vi "CG test stand DAQ main V3 LJ.vi"() -> ()   [LabVIEW 2023]
doc: "This example demonstrates how to read N channels of analog input from a LINX device."
uses:
  <vilib>/MakerHub/LINX/Public/Peripherals/Digital/Digital Write N Chans.vi
  <vilib>/MakerHub/LINX/Public/Peripherals/Analog/Analog Read N Chans.vi
  <vilib>/MakerHub/LINX/Private/Local IO/LinxDigitalWrite.vi
  <vilib>/MakerHub/LINX/Public/Utilities/Check Channel.vi
  <vilib>/MakerHub/LINX/Private/Local IO/LinxAnalogRead.vi
  <vilib>/MakerHub/LINX/Public/Utilities/Open Serial.vi
  <vilib>/MakerHub/LINX/Private/Utilties/Generate Error.vi
  <vilib>/Analysis/Matrix/Numeric/Conversions/Array To Matrix - RA.vi
  <vilib>/Utility/file.llb/Write Delimited Spreadsheet (DBL).vi
  <vilib>/MakerHub/LINX/LMH-LINX.lvlib
  <vilib>/Analysis/Matrix/NI_Matrix.lvlib
panel:
  in  "EIO Analog Enable":bool[](array[boolean])=[FALSE, FALSE, FALSE, FALSE, FALSE, FALSE, FALSE, FALSE]
  in  "FIO Analog Enable":bool[](array[boolean])=[FALSE, FALSE, FALSE, FALSE, FALSE, FALSE, FALSE, FALSE]
  in  "?":bool
  in  "Path":path
  out "Full filepath":string
  in  "File extension":string
  in  "Filename":string
  in  "Cal Value":dbl
  out "Time":timestamp
  out "Filewriting Error":errorcluster
  in  "FIO6":bool
  in  "FIO7":bool
  in  "DAC0":dbl format="%.4f"
  in  "Serial Port":refnum<visa-resource-name>
  out "LabJack Error":string
  in  "Device Selector":bool
  out "LABJACK U3 Error":errorcluster
  in  "Stop Button":bool
  in  "?":T1(tab)
  out "A0 B":dbl
  out "A0 X1":dbl
  out "A0 X2":dbl
  out "A0 X3":dbl
  out "A0 scaled":dbl
  out "A0_Instrumentlabel":dbl
  out "A0_Voltage":dbl
  out "A1":dbl
  out "A1_Voltage":dbl
  out "A2":dbl
  out "A2_Voltage":dbl
  out "A3":dbl
  out "A3_Voltage":dbl
  out "A1_Instrumentlabel":string
  out "A2_Instrumentlabel":string
  out "A3_Instrumentlabel":string
  out "A0_Instrumentlabel 2":string
  out "A2 B":dbl caption="A0 B"
  out "A2 X3":dbl caption="A0 X3"
  out "A2 X2":dbl caption="A0 X2"
  out "A2 X1":dbl caption="A0 X1"
  out "A2 scaled":dbl caption="A0 scaled"
  out "A3 B":dbl caption="A0 B"
  out "A3 X3":dbl caption="A0 X3"
  out "A3 X2":dbl caption="A0 X2"
  out "A3 X1":dbl caption="A0 X1"
  out "A3 scaled":dbl caption="A0 scaled"
  out "A4":dbl
  out "A4_Voltage":dbl
  out "A4_Instrumentlabel":string
  out "A4 X3":dbl caption="A0 X3"
  out "A4 X2":dbl caption="A0 X2"
  out "A4 X1":dbl caption="A0 X1"
  out "A4 B":dbl caption="A0 B"
  out "A4 scaled":dbl caption="A0 scaled"
  out "A4 2":dbl
  out "A5_Voltage":dbl
  out "A4_Instrumentlabel 2":string
  out "A5 B":dbl caption="A0 B"
  out "A5 X3":dbl caption="A0 X3"
  out "A5 X2":dbl caption="A0 X2"
  out "A5 X1":dbl caption="A0 X1"
  out "A5 scaled":dbl caption="A0 scaled"
  out "A2 scaled 2":dbl caption="A0 scaled"
  out "A2 X1 2":dbl caption="A0 X1"
  out "A2 X2 2":dbl caption="A0 X2"
  out "A2 X3 2":dbl caption="A0 X3"
  out "A2 B 2":dbl caption="A0 B"
  in  "?":string
  in  "Analog Port":dbl
  out "PLOT 2":dbl(graph)
  in  "?":string
  in  "Analog Port":dbl
  out "PLOT 1":dbl(graph)
  in  "Analog Port":dbl
  in  "?":string
  out "PLOT 3":dbl(graph)
  in  "Analog Port":dbl
  in  "?":string
  out "PLOT 4":dbl(graph)
  out "PT3":dbl
  out "TM-DEV-RES":dbl
  out "TM3":dbl
  out "TM2":dbl
  out "TM1":dbl
  out "PT1":dbl
  in  "Tare":dbl
  in  "Port":dbl
  out "Measured Load":dbl
  out "Loadcell Voltage":dbl
  in  "?":bool
  # "."
  # "HOW TO USE THIS SOFTWARE"
  # "1. Select the DAQ device you are using\n2. If you are using Arduino, select the COM port you are using\n3. Start the software by pressing CTRL+R"
  # "Analog Inputs"
  # "X1*V^1+X2*V^2+X3*V^3+B"
  # "Analog Port"
  # "Voltage In"
  # "X3"
  # "X2"
  # "X1"
  # "B"
  # "Instrument name"
  # "Scaled Value"
  # "F"
  # "psi"
  # "F"
  # "psi"
  # "F"
  # "psi"
  # "V"
  # "g"
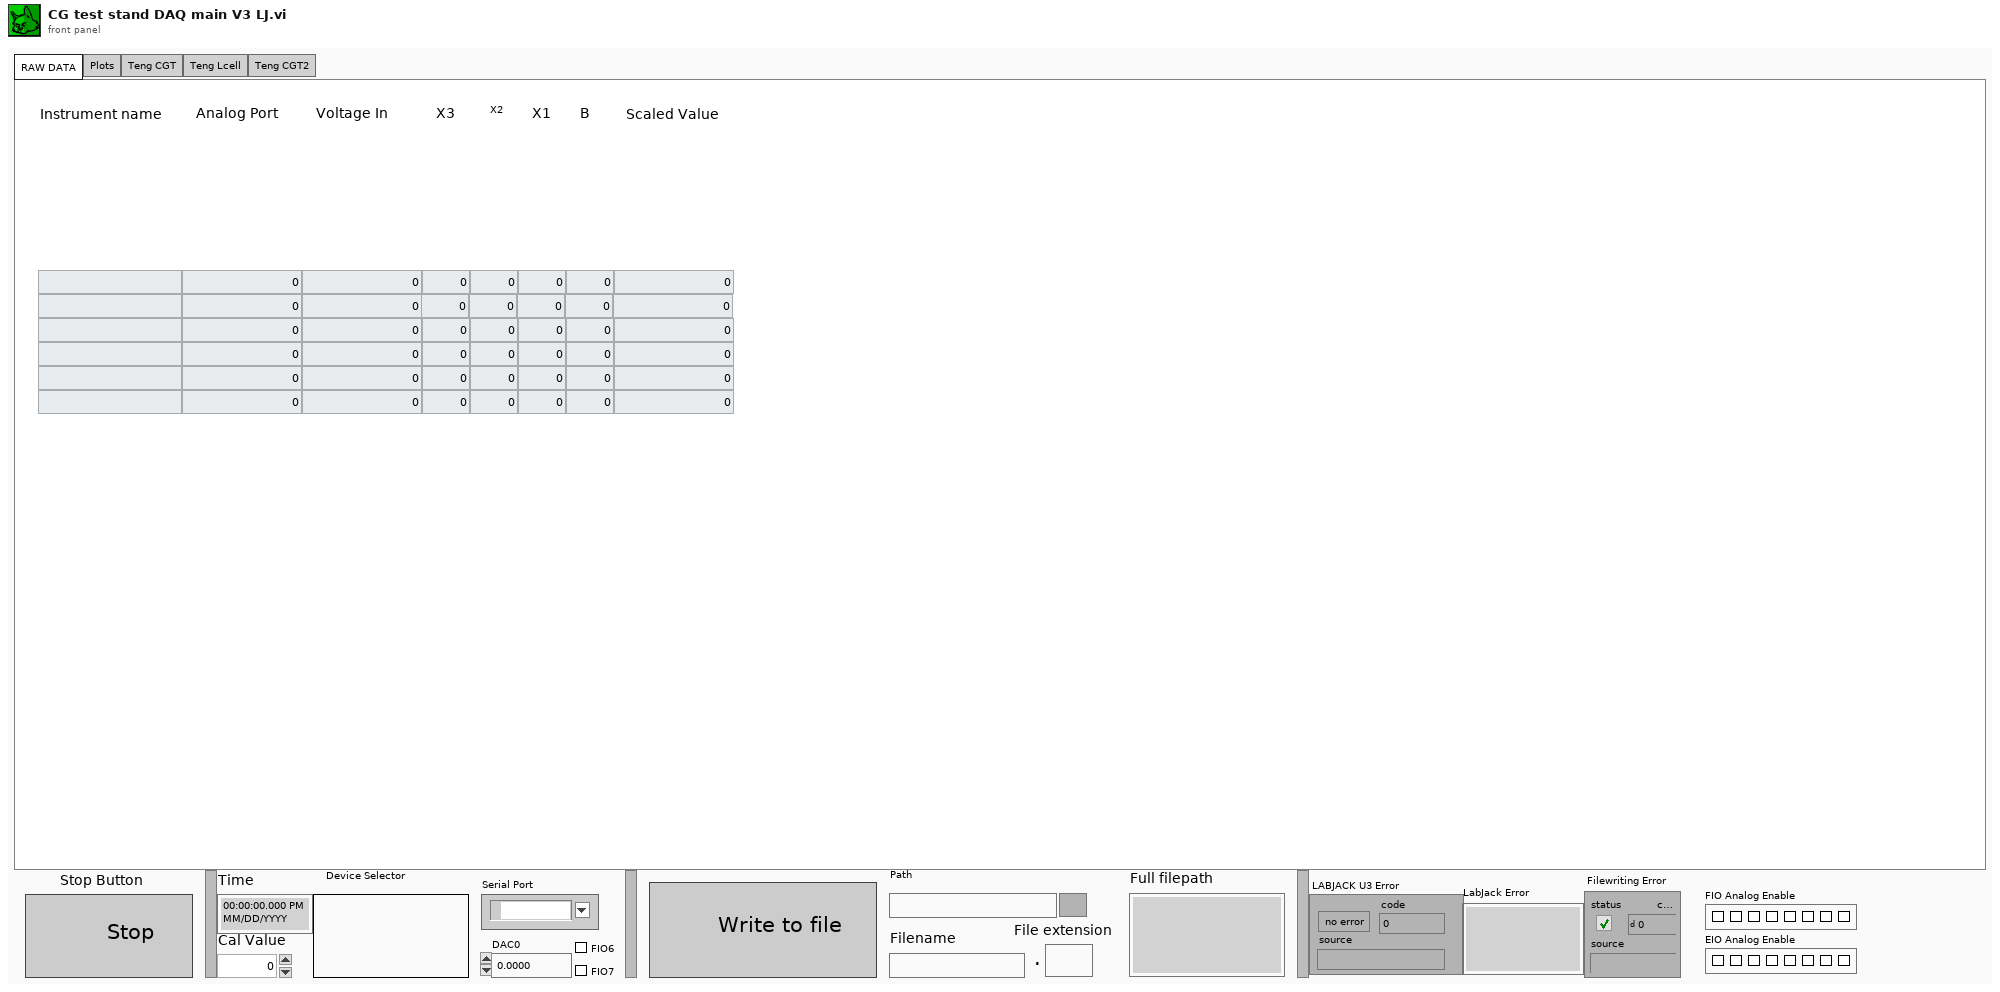
[diagram p1: front panel]
types:
  T1 = enum32{"RAW DATA", "Plots", "Teng CGT", "Teng Lcell", "Teng CGT2"}
  T2 = typedef "LMH-LINX.lvlib/LINX Ref.ctl" = cluster{"IO":T3, "Interface":T4, "LINX Device Config":T5}
  T3 = typedef "LMH-LINX.lvlib/Platform.ctl" = enum16{"Remote", "Local"}
  T4 = typedef "LMH-LINX.lvlib/Interface.ctl" = enum16{"Serial", "TCP"}
  T5 = typedef "LMH-LINX.lvlib/Device.lvlib/LINX Device Config.ctl" = cluster{"Interface":T4, "COM Port":refnum<visa-resource-name>, "TCP Configuration":T6, "Device Family":u8, "Device ID":u8, "Device Name":string, "TCP Ref":refnum<k5>, "Channels":T7}
  T6 = typedef "LMH-LINX.lvlib/Device.lvlib/TCP Config.ctl" = cluster{"IP Address":string, "Port":u16}
  T7 = typedef "LMH-LINX.lvlib/Channels.ctl" = cluster{"DI":u8[], "DO":u8[], "AI":u8[], "AO":u8[], "PWM":u8[], "QE":u8[], "UART":u8[], "I2C 2":u8[], "SPI":u8[], "CAN":u8[], "Servo":u8[], "AI Ref (V)":dbl, "AI Resolution (Bits)":u8, "AO Ref (V)":dbl, "AO Resolution (Bits)":u8}
  T8 = typedef "NI_Matrix.lvlib/RealMatrix.ctl" = dbl[][]
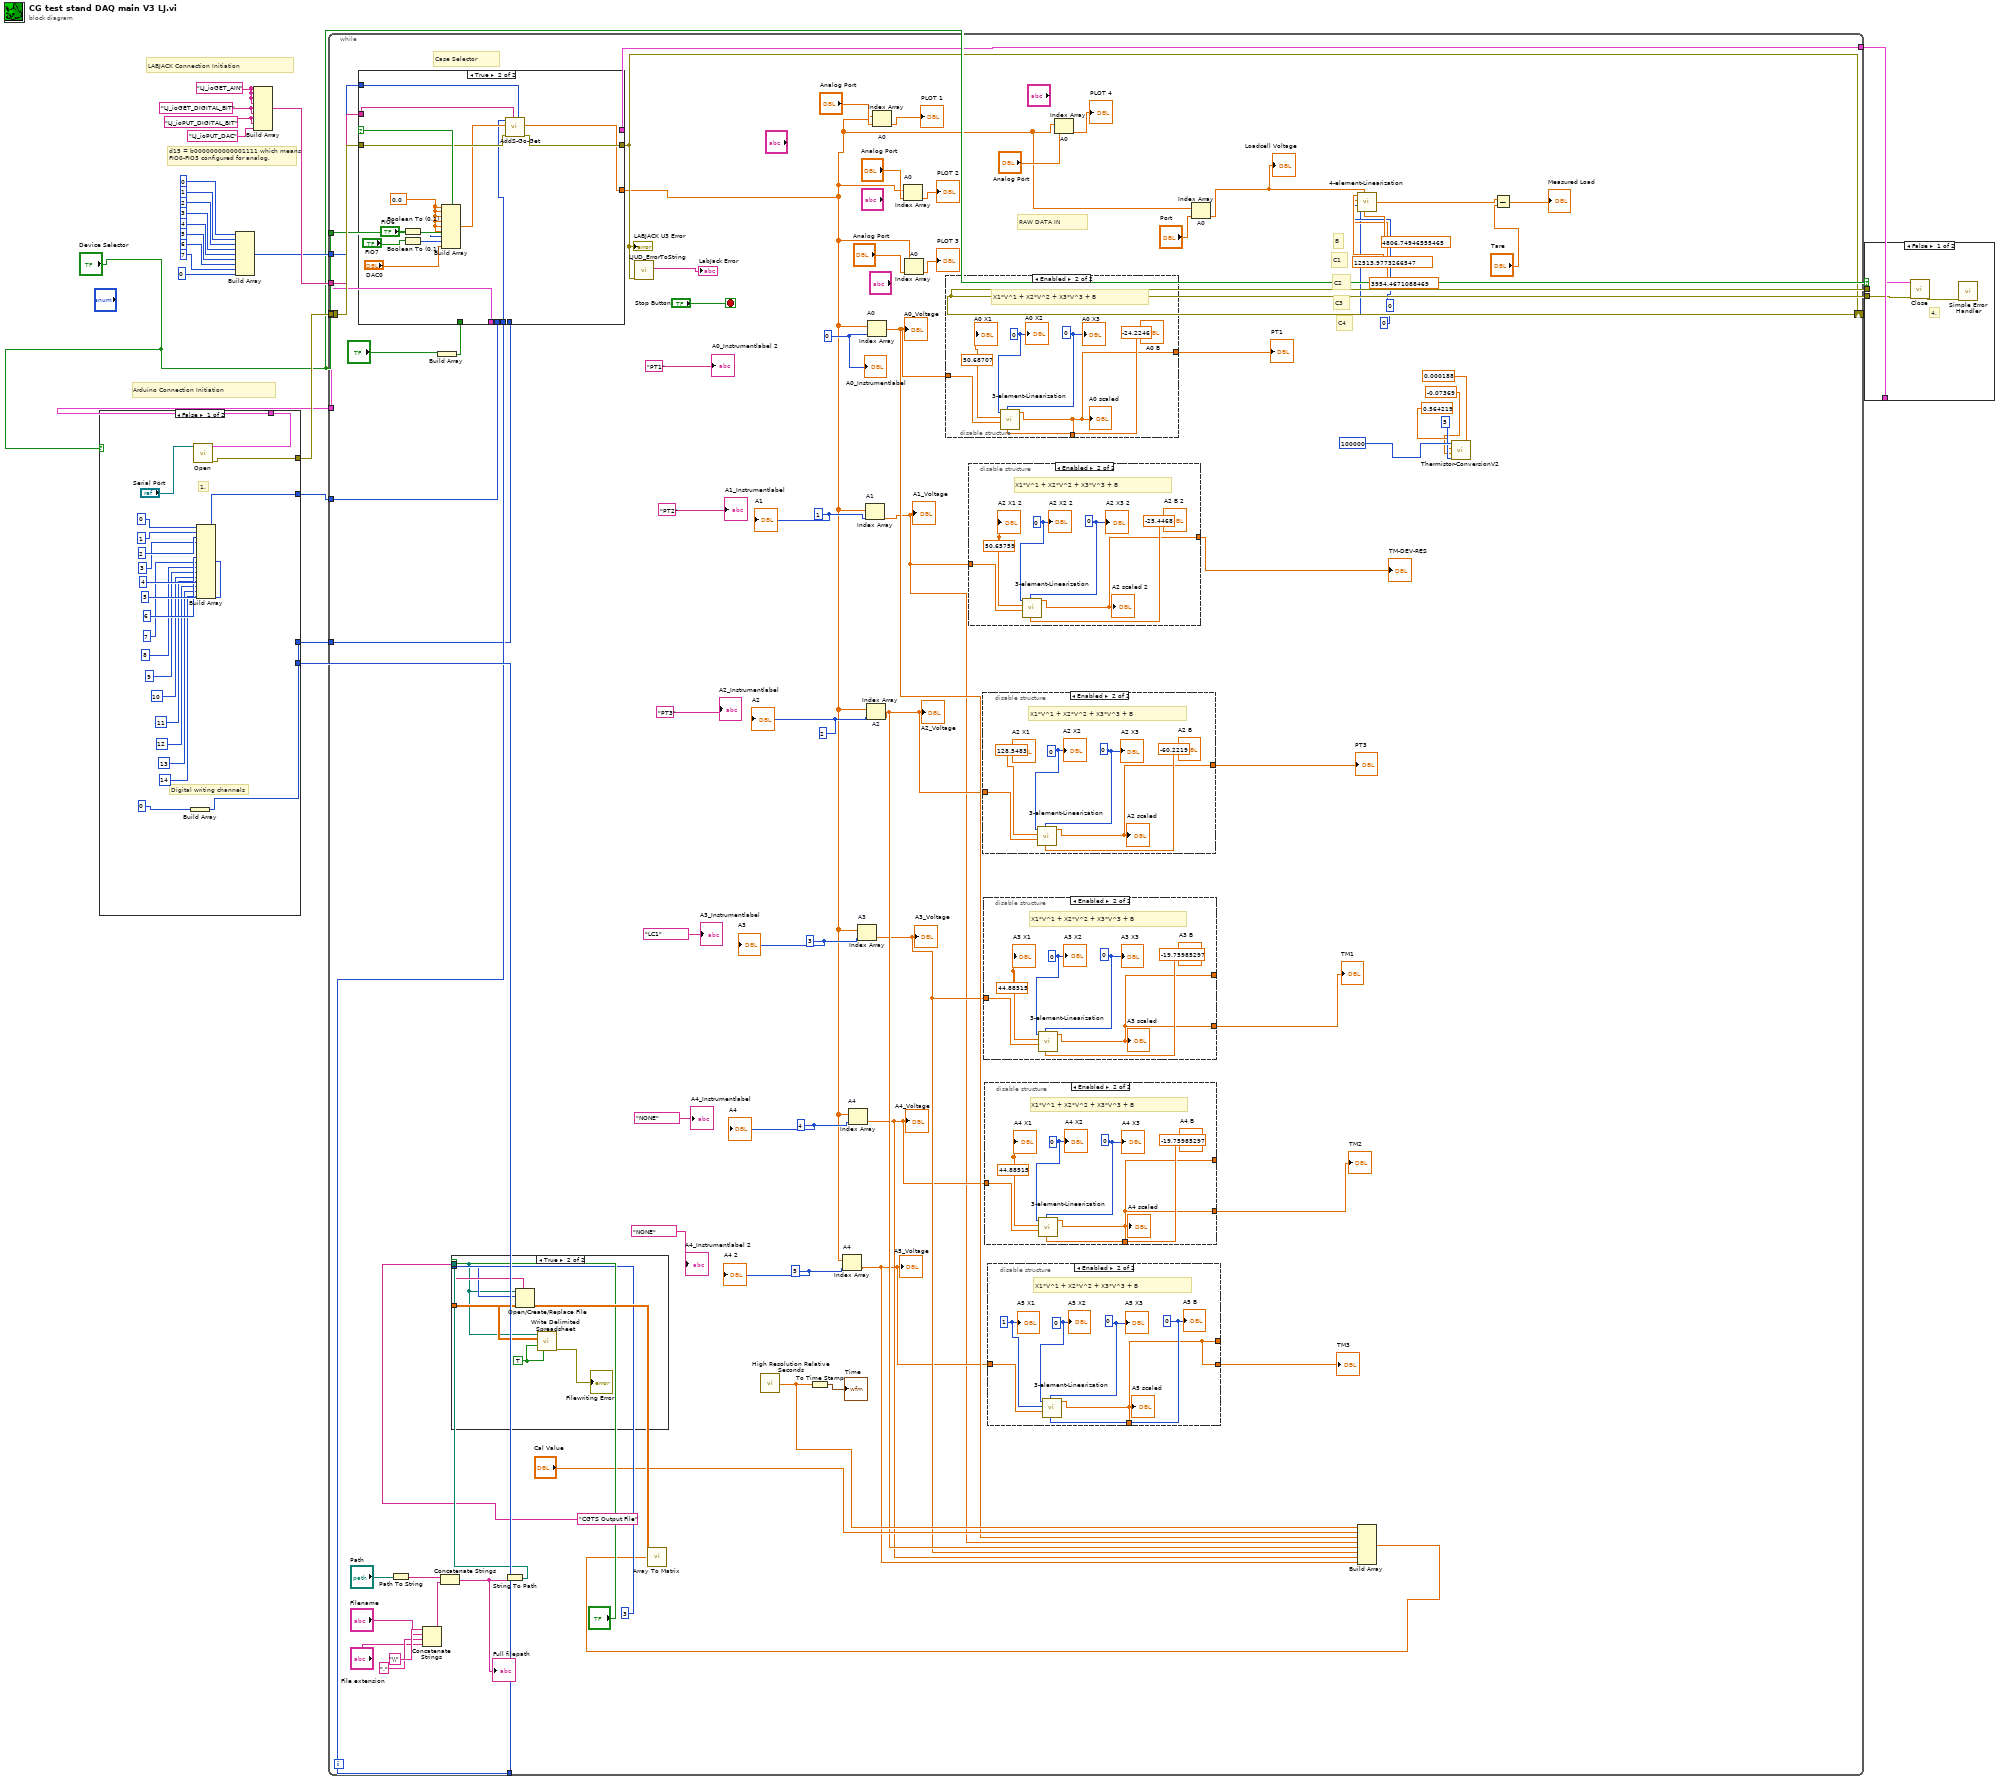
[diagram p0: block diagram]
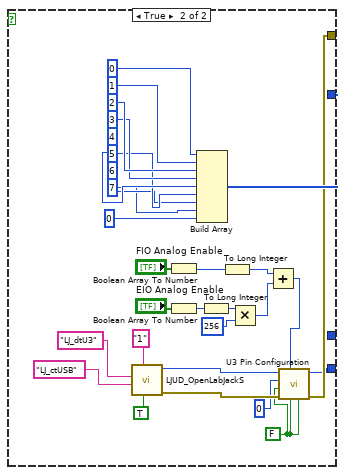
[diagram p3: hidden frame]
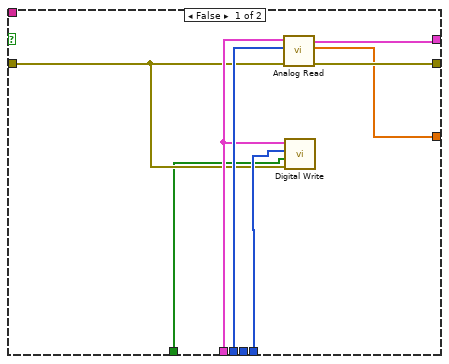
[diagram p11: hidden frame]
diagram:
  w21 = "LJ_ioPUT_DIGITAL_BIT" ("IOType")
  w23 = "LJ_ioGET_AIN" ("IOType")
  w22 = "LJ_ioGET_DIGITAL_BIT" ("IOType")
  # "Arduino Connection Initiation"
  # "LABJACK Connection Initiation"
  # "d15 = b0000000000001111 which means\nFIO0-FIO3 configured for analog."
  n1 = case shown="False" "Device Selector" {
    tunnel: [w38 w55] -> w19
    tunnel: [w37 _] -> w18
    tunnel: [w36 w64] -> w17
    tunnel: [_ w54] -> w3
    tunnel: [w33 _] -> w1
    frame False {
      # "Digital writing channels"
      # "1."
      n2 = Build Array(0) -> (w33:i32[])
      n3 = call-poly <vilib>:"Open.vi"("Serial Port"="Serial Port") -> ("Error Out"=w38:errorcluster, "LINX Resource"=w37:T2)  [unwired: 8 in, 1 out]
      n4 = Build Array(0, 1, 2, 3, 4, 5, 6, 7, 8, 9, 10, 11, 12, 13, 14) -> (w36:i32[])
    }
    frame True {
      w56 = FALSE ("Enable DAC1")
      n5 = call <vilib>:"LJUD_OpenLabJackS.vi"("FirstFound"=TRUE, "Address"="1", "ConnectionType"="LJ_ctUSB", "DeviceType"="LJ_dtU3") -> ("error out"=w59:errorcluster, "Handle"=w58:i32)  [unwired: 5 in, 1 out]
      n6 = Boolean Array To Number(Boolean array="FIO Analog Enable") -> (number=w49:u32)
      n7 = Boolean Array To Number(Boolean array="EIO Analog Enable") -> (number=w48:u32)
      n8 = Build Array(0, 1, 2, 3, 4, 5, 6, 7, 0) -> (w64:i32[])
      n9 = To Long Integer(number=w48) -> (32bit integer=w50:i32)
      n10 = To Long Integer(number=w49) -> (32bit integer=w47:i32)
      n11 = Multiply(x=w50, y=256) -> (x*y=w46:i32)
      n12 = Add(x=w47, y=w46) -> (x+y=w45:i32)
      n13 = call <vilib>:"U3 Pin Configuration.vi"("Enable Counter1"=w56, "Enable Counter0"=w56, "FIO/EIO Analog Enable"=w45, "error in"=w59, "Enable DAC1"=w56, "Number of Timers Enabled"=u8 0, "Handle In"=w58) -> ("error out"=w55:errorcluster, "Handle Out"=w54:i32)  [unwired: 3 in]
    }
  }
  n14 = Build Array(0, 1, 2, 3, 4, 5, 6, 7, 0) -> (w6:i32[])
  n15 = Build Array(w23, w23, w23, w23, w22, w22, w21, w21, "LJ_ioPUT_DAC" ("IOType")) -> (w16:string[])
  n16 = while {
    tunnel: w19 -> [w152]
    tunnel: w18 -> [w151]
    tunnel: [w150] -> w4
    shift-right: [w142] -> w5
    shift-left: _ -> [_]
    tunnel: w17 -> [w149]
    tunnel: "Device Selector" -> [w148]
    tunnel: w16 -> [w147]
    tunnel: w6 -> [w146]
    tunnel: w3 -> [w144]
    tunnel: w1 -> [w76]
    stop <- "Stop Button" stop-if-true
    w117 = 5
    w119 = 4
    w139 = 3
    w138 = 2
    w140 = 1
    w141 = 0
    # "B"
    # "C4"
    # "C3"
    # "C2"
    # "C1"
    # "RAW DATA IN"
    # "Case Selector"
    n17 = Path To String(path="Path") -> (string=w126:string)
    n18 = Concatenate Strings("\\", "Filename", ".", "File extension") -> (w125:string)
    n19 = Build Array("?") -> (w74:bool[])
    n20 = case shown="True" w148 {
      tunnel: [w202 w214] -> w142
      tunnel: w152 -> [w196 w215]
      tunnel: w151 -> [w198 _]
      tunnel: [w201 _] -> w150
      tunnel: w149 -> [w200 _]
      tunnel: w147 -> [_ w208]
      tunnel: w146 -> [_ w207]
      tunnel: [w199 w204] -> w102
      tunnel: w144 -> [_ w203]
      tunnel: w76 -> [w197 _]
      tunnel: w74 -> [w195 _]
      frame False {
        n21 = call-poly <vilib>:"Analog Read.vi"("Error In"=w196, "AI Channel(s)"=w200, "LINX Resource"=w198) -> ("Error Out"=w202:errorcluster, "Voltages"=w199:dbl[], "LINX Resource"=w201:T2)  [unwired: 5 in, 1 out]
        n22 = call-poly <vilib>:"Digital Write.vi"("Error In"=w196, "Values"=w195, "DO Channels"=w197, "LINX Resource"=w198) -> ()  [unwired: 6 in, 2 out]
      }
      frame True {
        w206 = 0.0 ("Input Element")
        n23 = Boolean To (0,1)(Boolean="FIO6") -> (0, 1=w213:i16)
        n24 = Boolean To (0,1)(Boolean="FIO7") -> (0, 1=w212:i16)
        n25 = Build Array(w206, w206, w206, w206, w206, w206, w213, w212, "DAC0") -> (w209:dbl[])
        n26 = call <vilib>:"AddS-Go-Get.vi"("Channels"=w207, "IOTypes"=w208, "error in"=w215, "Values Write"=w209, "Handle In"=w203) -> ("error out"=w214:errorcluster, "Values Read"=w204:dbl[])  [unwired: 4 in, 1 out]
      }
    }
    "LABJACK U3 Error" <- w142
    n27 = Concatenate Strings(w126, w125) -> (w124:string)
    "Full filepath" <- w124
    n28 = String To Path(string=w124) -> (path=w123:path)
    n29 = call <vilib>:"LJUD_ErrorToString.vi"("error in"=w142) -> ("String"=→"LabJack Error":string)  [unwired: 10 in]
    n30 = call <vilib>:"High Resolution Relative Seconds.vi"() -> ("relative seconds"=w84:dbl)
    n31 = To Time Stamp(1:w84) -> (0:→"Time":timestamp)
    n32 = Index Array "A4"(array=w102, index=w117) -> (element=w79:dbl)
    "A5_Voltage" <- w79
    n33 = Index Array "A4"(array=w102, index=w119) -> (element=w80:dbl)
    "A4_Voltage" <- w80
    n34 = Index Array "A3"(array=w102, index=w139) -> (element=w81:dbl)
    "A3_Voltage" <- w81
    n35 = Index Array "A1"(array=w102, index=w140) -> (element=w78:dbl)
    "A1_Voltage" <- w78
    n36 = Index Array "A2"(array=w102, index=w138) -> (element=w82:dbl)
    "A2_Voltage" <- w82
    n37 = Index Array "A0"(array=w102, index=w141) -> (element=w83:dbl)
    "A0_Voltage" <- w83
    n38 = Index Array "A0"(array=w102, index="Analog Port") -> (element=→"PLOT 1":dbl)
    n39 = Index Array "A0"(array=w102, index="Analog Port") -> (element=→"PLOT 2":dbl)
    n40 = Index Array "A0"(array=w102, index="Analog Port") -> (element=→"PLOT 3":dbl)
    n41 = disable-structure shown="Enabled" {
      disable-tunnel: w83 -> [_ w194]
      disable-tunnel: [_ w189] -> _
      disable-tunnel: [_ w189] -> w113
      frame Disabled {
      }
      frame Enabled {
        w190 = -24.2246
        w193 = 0
        w192 = 0
        w191 = 50.68707
        # "X1*V^1 + X2*V^2 + X3*V^3 + B"
        n42 = call "3-element-Linearization.vi"("B"=w190, "C3"=w193, "Voltage in"=w194, "C1"=w191, "C2"=w192) -> ("Scaled value"=w189:dbl)  [unwired: 6 in]
        "A0 scaled" <- w189
        "A0 X1" <- w191
        "A0 X2" <- w192
        "A0 X3" <- w193
        "A0 B" <- w190
      }
    }
    "PT1" <- w113
    n43 = disable-structure shown="Enabled" {
      disable-tunnel: w78 -> [_ w158]
      disable-tunnel: [_ w153] -> w77
      frame Disabled {
      }
      frame Enabled {
        w154 = -25.4468
        w157 = 0
        w156 = 0
        w155 = 50.65759
        # "X1*V^1 + X2*V^2 + X3*V^3 + B"
        n44 = call "3-element-Linearization.vi"("B"=w154, "C3"=w157, "Voltage in"=w158, "C1"=w155, "C2"=w156) -> ("Scaled value"=w153:dbl)  [unwired: 6 in]
        "A2 scaled 2" <- w153
        "A2 X1 2" <- w155
        "A2 X2 2" <- w156
        "A2 X3 2" <- w157
        "A2 B 2" <- w154
      }
    }
    "TM-DEV-RES" <- w77
    n45 = disable-structure shown="Enabled" {
      disable-tunnel: w82 -> [_ w188]
      disable-tunnel: [_ w183] -> w112
      frame Disabled {
      }
      frame Enabled {
        w184 = -60.2219
        w187 = 0
        w186 = 0
        w185 = 128.5483
        # "X1*V^1 + X2*V^2 + X3*V^3 + B"
        n46 = call "3-element-Linearization.vi"("B"=w184, "C3"=w187, "Voltage in"=w188, "C1"=w185, "C2"=w186) -> ("Scaled value"=w183:dbl)  [unwired: 6 in]
        "A2 scaled" <- w183
        "A2 X1" <- w185
        "A2 X2" <- w186
        "A2 X3" <- w187
        "A2 B" <- w184
      }
    }
    "PT3" <- w112
    n47 = disable-structure shown="Enabled" {
      disable-tunnel: w81 -> [_ w182]
      disable-tunnel: [_ w177] -> _
      disable-tunnel: [_ w177] -> w114
      frame Disabled {
      }
      frame Enabled {
        w178 = -19.75985297
        w181 = 0
        w180 = 0
        w179 = 44.88515
        # "X1*V^1 + X2*V^2 + X3*V^3 + B"
        n48 = call "3-element-Linearization.vi"("B"=w178, "C3"=w181, "Voltage in"=w182, "C1"=w179, "C2"=w180) -> ("Scaled value"=w177:dbl)  [unwired: 6 in]
        "A3 scaled" <- w177
        "A3 X1" <- w179
        "A3 X2" <- w180
        "A3 X3" <- w181
        "A3 B" <- w178
      }
    }
    "TM1" <- w114
    n49 = disable-structure shown="Enabled" {
      disable-tunnel: w80 -> [_ w170]
      disable-tunnel: [_ w165] -> _
      disable-tunnel: [_ w165] -> _
      disable-tunnel: [_ w165] -> w115
      frame Disabled {
      }
      frame Enabled {
        w166 = -19.75985297
        w169 = 0
        w168 = 0
        w167 = 44.88515
        # "X1*V^1 + X2*V^2 + X3*V^3 + B"
        n50 = call "3-element-Linearization.vi"("B"=w166, "C3"=w169, "Voltage in"=w170, "C1"=w167, "C2"=w168) -> ("Scaled value"=w165:dbl)  [unwired: 6 in]
        "A4 scaled" <- w165
        "A4 X1" <- w167
        "A4 X2" <- w168
        "A4 X3" <- w169
        "A4 B" <- w166
      }
    }
    "TM2" <- w115
    n51 = disable-structure shown="Enabled" {
      disable-tunnel: w79 -> [_ w164]
      disable-tunnel: [_ w159] -> _
      disable-tunnel: [_ w159] -> _
      disable-tunnel: [_ w159] -> w111
      frame Disabled {
      }
      frame Enabled {
        w160 = 0
        w163 = 0
        w162 = 0
        w161 = 1
        # "X1*V^1 + X2*V^2 + X3*V^3 + B"
        n52 = call "3-element-Linearization.vi"("B"=w160, "C3"=w163, "Voltage in"=w164, "C1"=w161, "C2"=w162) -> ("Scaled value"=w159:dbl)  [unwired: 6 in]
        "A5 scaled" <- w159
        "A5 X1" <- w161
        "A5 X2" <- w162
        "A5 X3" <- w163
        "A5 B" <- w160
      }
    }
    "TM3" <- w111
    n53 = Index Array "A0"(array=w102, index="Analog Port") -> (element=→"PLOT 4":dbl)
    n54 = Index Array "A0"(array=w102, index="Port") -> (element=w95:dbl)
    "Loadcell Voltage" <- w95
    n55 = call "4-element-Linearization.vi"("B"=4806.74946555465, "Voltage in"=w95, "C4"=0, "C3"=0, "C2"=3954.4671088469, "C1"=12513.9773266547) -> ("Scaled value"=w94:dbl)
    n56 = Build Array(w84, "Cal Value", w83, w78, w82, w81, w80, w79) -> (w86:dbl[])
    n57 = call-poly <vilib>:"Array To Matrix.vi"("Real 1D Array"=w86) -> ("Real Matrix (Column Vector)"=w133:T8)
    n58 = case shown="True" "?" {
      tunnel: [_ w171] -> _
      tunnel: w133 -> [_ w172]
      tunnel: "CGTS Output File" -> [_ w176]
      tunnel: 3 -> [_ w175]
      tunnel: w123 -> [_ w171]
      frame False {
      }
      frame True {
        w173 = TRUE
        n59 = Open/Create/Replace File(file path (use dialog)=w171, prompt=w176, operation (0:open)=w175) -> ()  [unwired: 3 in, 3 out]
        n60 = call-poly <vilib>:"Write Delimited Spreadsheet.vi"("file path (dialog if empty)"=w171, "2D data"=w172, "append to file? (new file:F)"=w173, "transpose? (no:F)"=w173) -> ("error out"=→"Filewriting Error":errorcluster)  [unwired: 10 in, 1 out]
      }
    }
    n61 = call "Thermistor-ConversionV2.vi"("Resistor"=100000, "A"=0.564219, "B"=-0.07369, "Input voltage"=5, "C"=0.000188) -> ()  [unwired: 1 in, 1 out]
    n62 = Subtract(x=w94, y="Tare") -> (x-y=→"Measured Load":dbl)
    "A0_Instrumentlabel" <- w141
    "A1" <- w140
    "A2" <- w138
    "A3" <- w139
    "A1_Instrumentlabel" <- "PT2"
    "A2_Instrumentlabel" <- "PT3"
    "A3_Instrumentlabel" <- "LC1"
    "A0_Instrumentlabel 2" <- "PT1"
    "A4" <- w119
    "A4_Instrumentlabel" <- "NONE"
    "A4 2" <- w117
    "A4_Instrumentlabel 2" <- "NONE"
  }
  n63 = case shown="False" "Device Selector" {
    tunnel: w5 -> [_ _]
    tunnel: w5 -> [w216 _]
    tunnel: w4 -> [w217 _]
    frame False {
      # "4."
      n64 = call <vilib>:"Close.vi"("Error In"=w216, "LINX Resource"=w217) -> ("Error Out"=w218:errorcluster)  [unwired: 9 in]
      n65 = call <vilib>:"Simple Error Handler.vi"("error in (no error)"=w218) -> ()  [unwired: 4 in, 5 out]
    }
    frame True {
    }
  }
